vi "HW_QX_DAQ FGV.vi"(0 "DevListTree":refnum<vi>, 1 "Oper.":T3, 5 "ActiveModuTag":string, 7 "Paravalues[]":string[][](array[string]), 11 "error in":errorcluster caption="错误输入") -> (4 "ActiveCFG":T1, 6 "UsedQXcfg":T1[](array[typedef]), 8 "data":dbl[][](array[numeric]), 10 "ChanPara.CHName":string[](array[string]), 13 "SampRate":dbl, 14 "T0":timestamp, 15 "error out":errorcluster caption="错误输出")   [LabVIEW 2016]
uses:
  QX DAQ FGV Operations.ctl
  Ctrls/HardWare _ Module Configuration.ctl
panel:
  out "data":waveform(dbl)[](array[waveform])
  in  "CFGinTree":T2
  in  "QXcfg in":T1[](array[typedef])
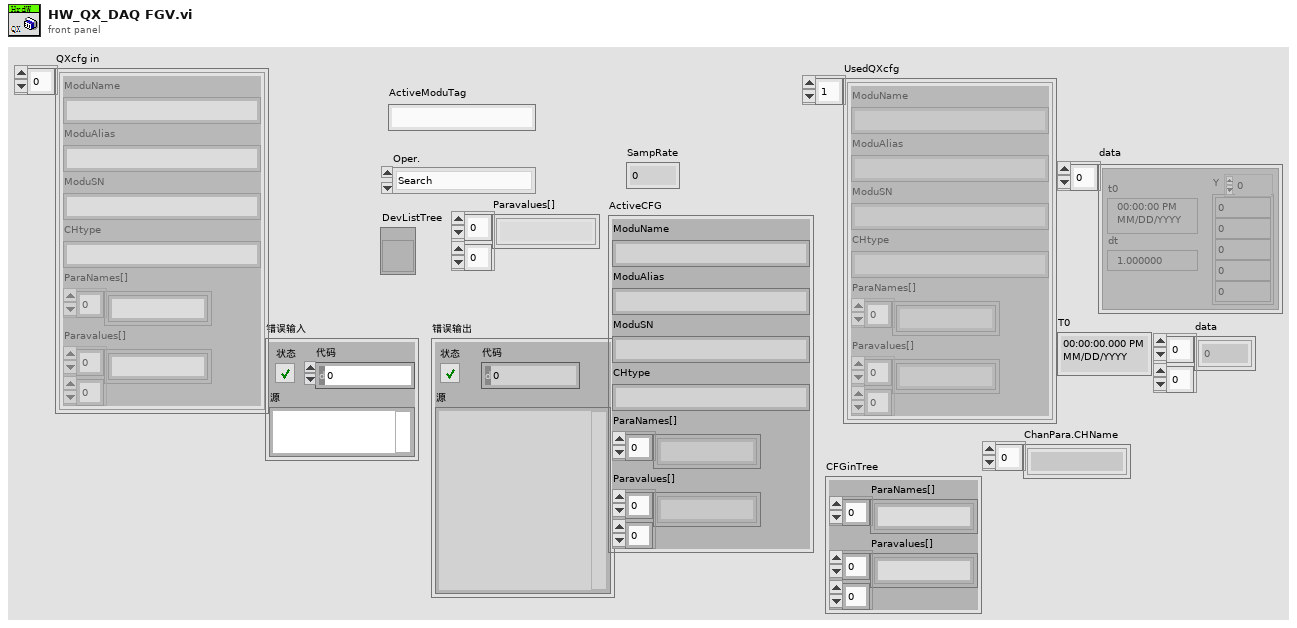
[diagram p1: front panel]
types:
  T1 = typedef "HardWare _ Module Configuration.ctl" = cluster{"ModuName":string, "ModuAlias":string, "ModuSN":string, "CHtype":string, "ParaNames[]":string[], "Paravalues[]":string[][]}
  T2 = cluster{"ParaNames[]":string[], "Paravalues[]":string[][]}
  T3 = typedef "QX DAQ FGV Operations.ctl" = enum16{"Search", "ReadCFG", "UpdateTempCFG", "DownloadCFG", "StartDAQ", "RunDAQ", "StopDAQ", "DisConnect"}
  T4 = typedef "QX Module Info.ctl" = cluster{"ModuName":string, "ModuSN":string, "ModuIP":string, "Port":i32, "ChType":string, "ChanNames[]":string[]}
  T5 = cluster{"QX DevInfo[]":T4[], "Devices":refnum<k24>[]}
  T6 = cluster{"ParaFolder":path, "SysCfg":path, "CHdef":path, "ModCfg":path, "DT Folder":path, "ErrorLog":path, "HBMDriverlicense":path}
  T7 = cluster{"ModuRef":refnum<k24>, "ChRef[]":refnum<k24>[]}[]
  T8 = typedef "HardWare _ Channel Configurations PopUp Type.ctl" = cluster{"Pop Type":T9, "PopValue":string}
  T9 = typedef "POP_Data Type.ctl" = enum16{"NO POPUP", "Unkown", "String", "Integer", "Float", "Color", "Boolean", "Ring", "Captioned String", "Captioned Integer", "Button Color", "2 Int Cluster", "4 Int Cluster", "6-Dbl Cluster", "Path", "Combox", "Time", "ShotCut String"}
  T10 = cluster{"ParaNames":string[], "DfltPara":string[], "Types":string[], "PopTypes":T8[]}
  T11 = typedef "HardWare _ Channel Parameters.ctl" = cluster{"CHType":string[], "CHName":string[], "CHAlias":string[], "Use":bool[], "Unit":string[], "SampleRate":dbl[], "FilterFreq":dbl[], "SlopeA":dbl[], "InterceptB":dbl[], "SampMax":dbl[], "SampMin":dbl[], "AlarmMax":dbl[], "AlarmMin":dbl[]}
  T12 = cluster{"AllInUsedChan[]":refnum<k24>[], "ChanPara":T11}
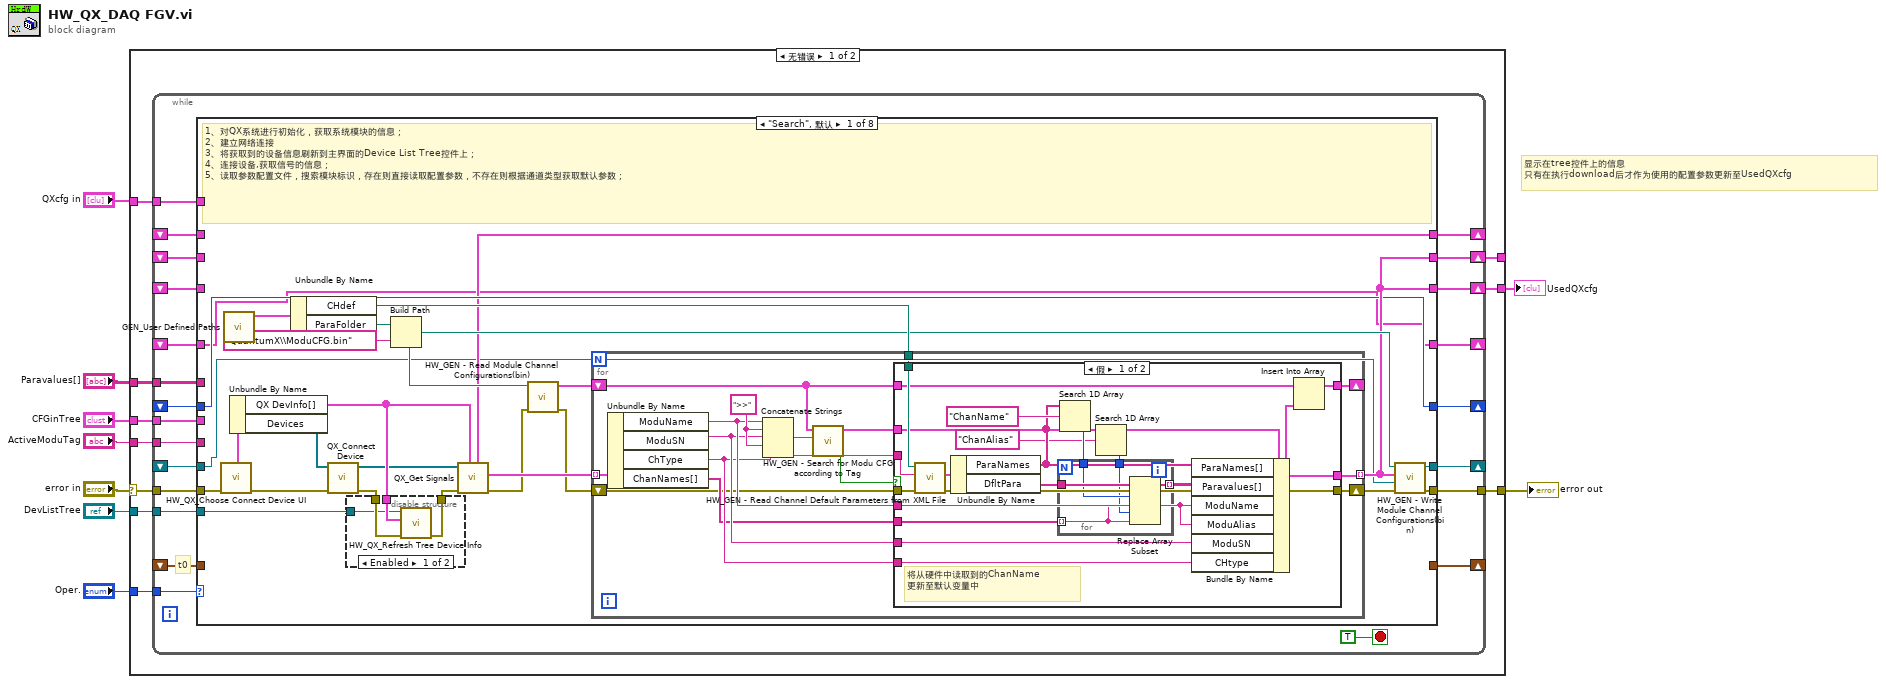
[diagram p0: block diagram]
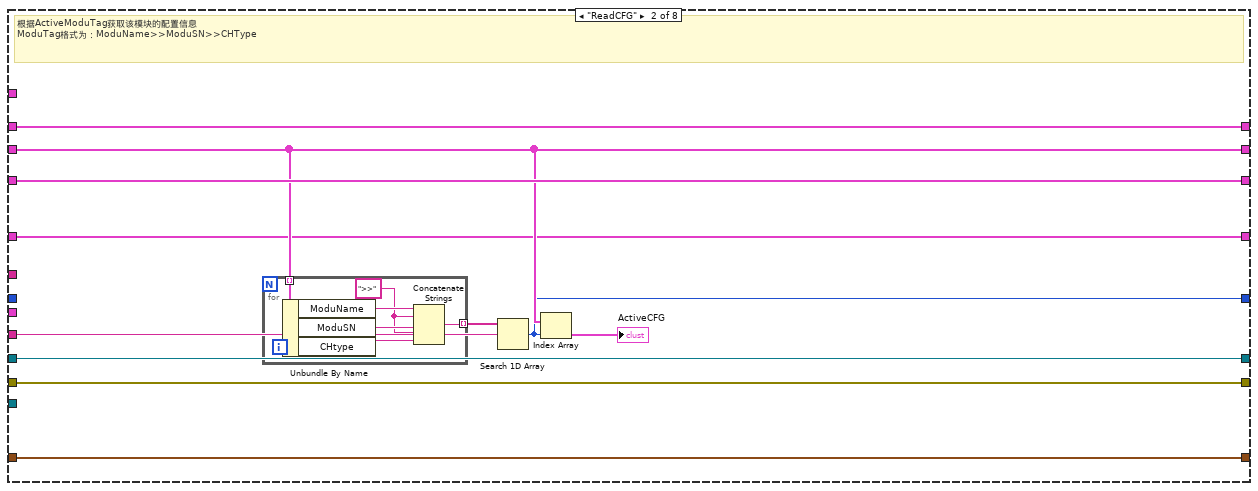
[diagram p4: hidden frame]
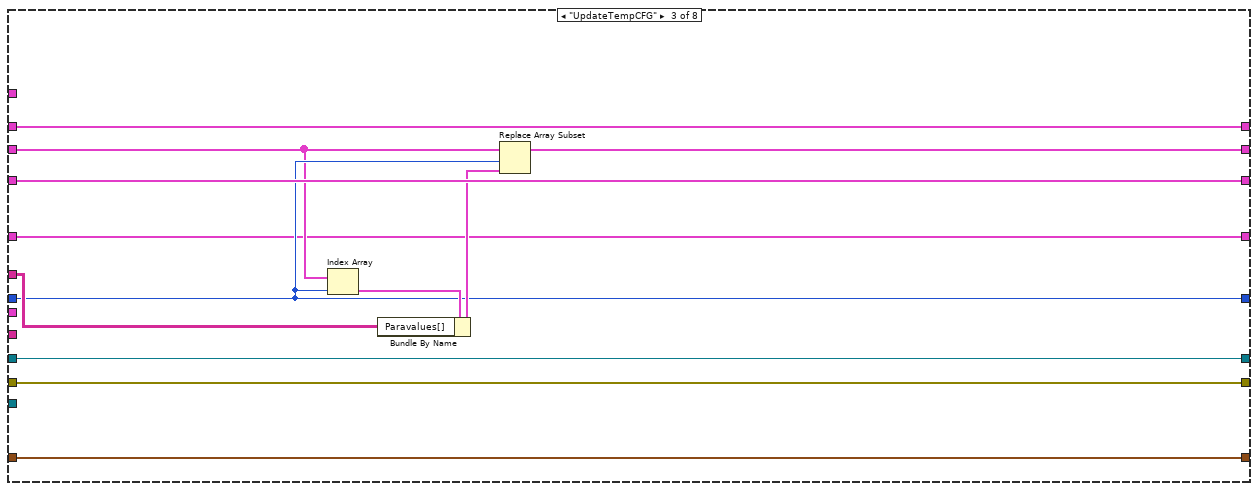
[diagram p5: hidden frame]
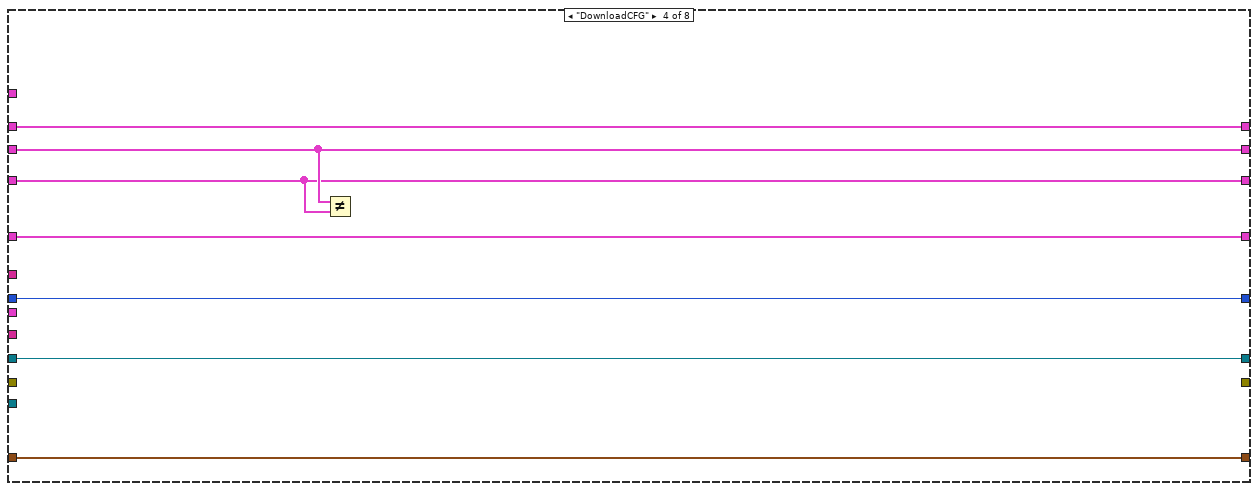
[diagram p6: hidden frame]
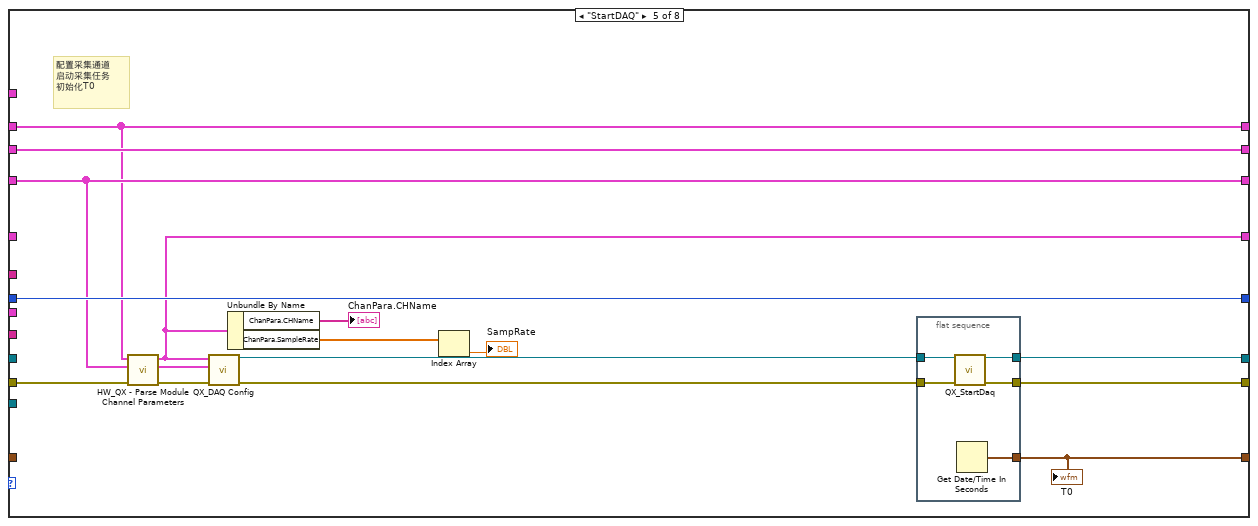
[diagram p7: hidden frame]
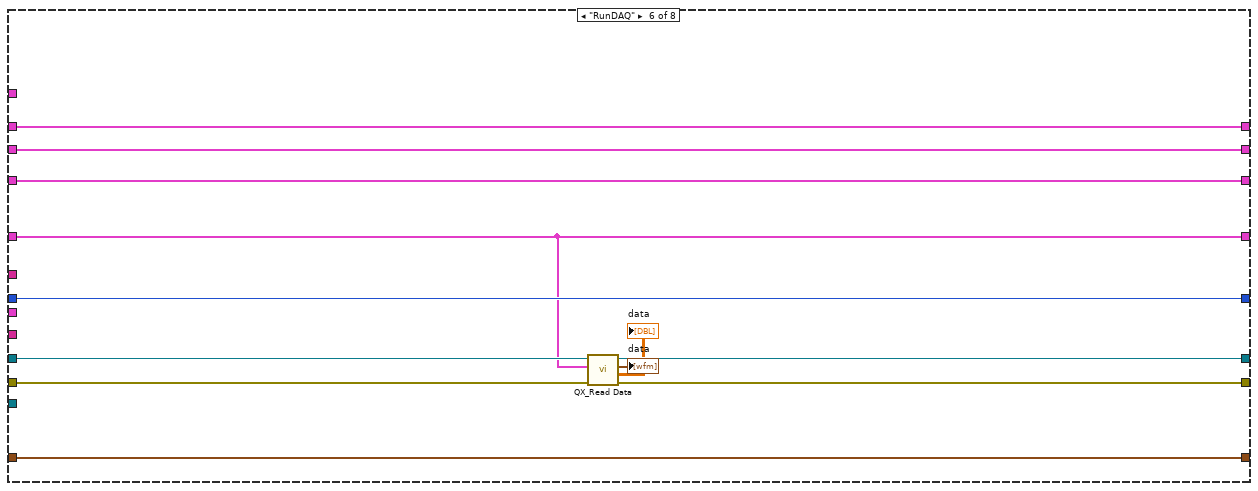
[diagram p8: hidden frame]
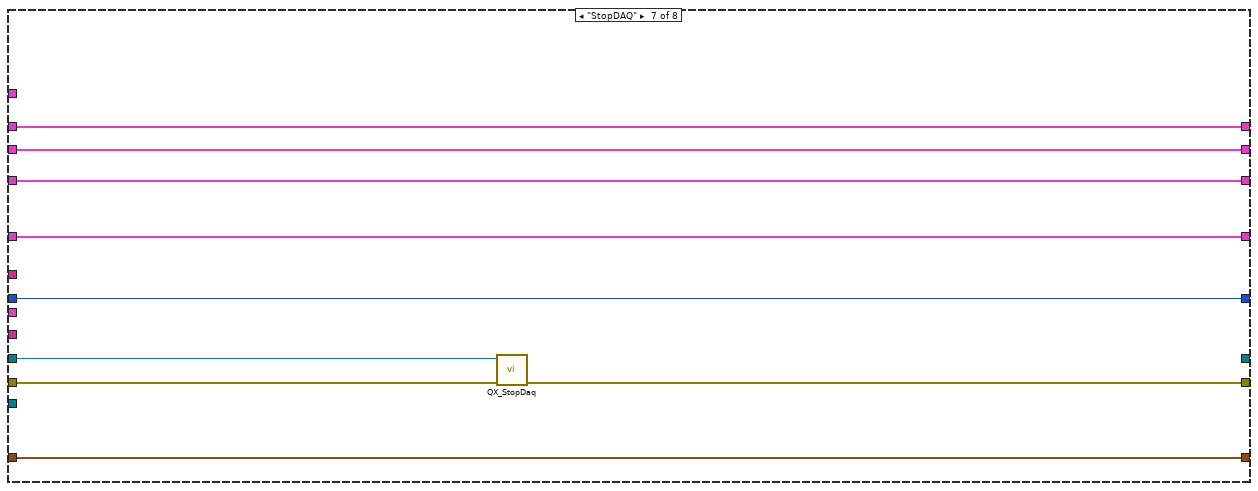
[diagram p9: hidden frame]
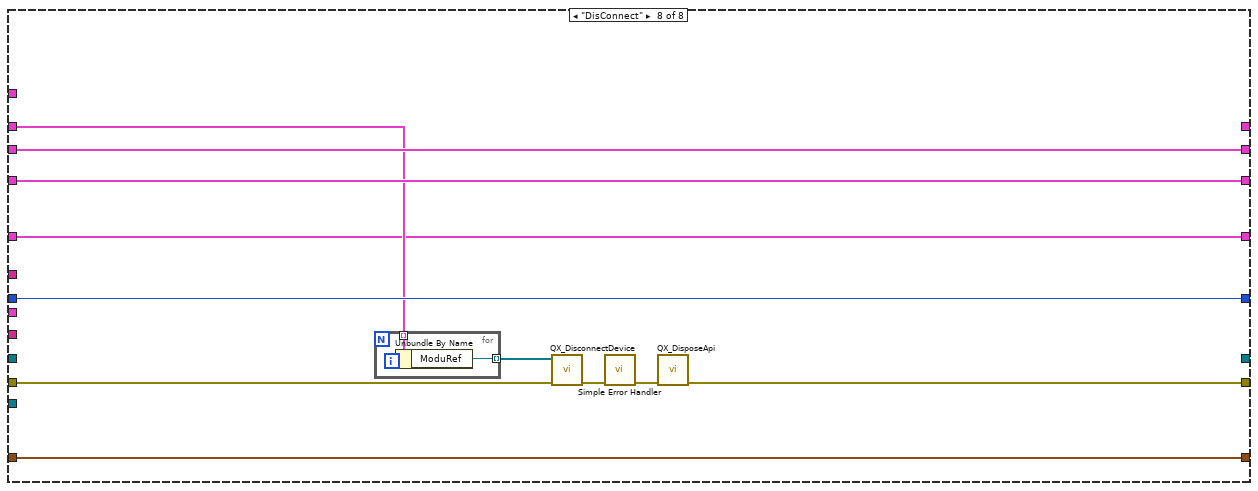
[diagram p10: hidden frame]
diagram:
  # "显示在tree控件上的信息\n只有在执行download后才作为使用的配置参数更新至UsedQXcfg"
  n1 = case shown="无错误" "error in" {
    selector: "error in" -> [w18 w207]
    tunnel: [w17 w207] -> w8
    tunnel: "Oper." -> [w19 _]
    tunnel: [w16 _] -> w6
    tunnel: "DevListTree" -> [w15 _]
    tunnel: "QXcfg in" -> [w14 _]
    tunnel: "ActiveModuTag" -> [w13 _]
    tunnel: [w12 _] -> _
    tunnel: "CFGinTree" -> [w11 _]
    tunnel: "Paravalues[]" -> [w10 _]
    frame No Error {
      n2 = while {
        tunnel: w19 -> [w41]
        tunnel: w18 -> [w40]
        tunnel: [w39] -> w17
        shift-right: [w38] -> _
        shift-left: _ -> [w37]
        shift-right: [w36] -> w16
        shift-left: _ -> [w35]
        tunnel: w15 -> [w34]
        tunnel: w14 -> [w33]
        tunnel: w13 -> [w32]
        shift-right: [w31] -> w12
        shift-left: _ -> [w30]
        tunnel: w11 -> [w29]
        shift-right: [w28] -> _
        shift-left: _ -> [w27]
        tunnel: w10 -> [w26]
        shift-right: [w25] -> _
        shift-left: _ -> [w24]
        shift-right: [w23] -> _
        shift-left: _ -> [w22]
        shift-right: [w21] -> _
        shift-left: _ -> [w20]
        stop <- TRUE stop-if-true
        # "t0"
        n3 = case shown="\"Search\", 默认" w41 {
          tunnel: w40 -> [w67 w125 w143 _ w158 w180 w187 w198]
          tunnel: [w58 w125 w143 _ w162 w177 w185 w196] -> w39
          tunnel: [_ w126 w144 w151 w167 w184 w193 w204] -> w38
          tunnel: w37 -> [_ w126 w144 w151 _ w184 w193 w204]
          tunnel: [w48 w122 w142 w145 w160 w181 w190 w203] -> w36
          tunnel: w35 -> [_ w122 w142 w145 w160 w181 w190 w203]
          tunnel: w34 -> [w53 _ _ _ _ _ _ _]
          tunnel: w33 -> [_ _ _ _ _ _ _ _]
          tunnel: w32 -> [_ w123 _ _ _ _ _ _]
          tunnel: [w48 w121 w136 w146 w165 w182 w191 w202] -> w31
          tunnel: w30 -> [_ w121 w137 w146 w165 w182 w191 w202]
          tunnel: w29 -> [_ _ _ _ _ _ _ _]
          tunnel: [w47 w120 w138 w150 w166 w183 w192 w201] -> w28
          tunnel: w27 -> [w47 _ w138 w150 w166 w183 w192 w201]
          tunnel: w26 -> [_ _ w140 _ _ _ _ _]
          tunnel: [w45 w118 w135 w149 w159 w176 w189 _] -> w25
          tunnel: w24 -> [_ w118 w135 w149 w159 w176 w189 w200]
          tunnel: [w44 w117 w134 w148 w161 w178 _ _] -> w23
          tunnel: w22 -> [w44 w117 w134 w148 _ w179 w186 _]
          tunnel: [w43 w116 w133 w147 w155 w175 w188 w194] -> w21
          tunnel: w20 -> [w43 w116 w133 w147 _ w175 w188 w194]
          frame "Search", Default {
            # "1、对QX系统进行初始化，获取系统模块的信息；\n2、建立网络连接\n3、将获取到的设备信息刷新到主界面的Device List Tree控件上；\n4、连接设备,获取信号的信息；\n5、读取参数配置文件，搜索模块标识，存在则直接读取配置参数，不存在则根据通道类型获取默认参数；"
            n4 = call "HW_QX_Choose Connect Device UI.vi"("error in"=w67) -> ("error out"=w66:errorcluster, "QX Dev"=w65:T5)  [unwired: 9 in]
            n5 = call "GEN_User Defined Paths.vi"() -> ("UserDefinedPath"=w63:T6)  [unwired: 11 in]
            n6 = Unbundle By Name(w65) -> ("QX DevInfo[]"=w54:T4[], "Devices"=w64:refnum<k24>[])
            n7 = Unbundle By Name(w63) -> ("CHdef"=w60:path, "ParaFolder"=w61:path)
            n8 = call "QX_Connect Device.vi"("error in"=w66, "Devices"=w64) -> ("error out"=w56:errorcluster, "Devices"=w46:refnum<k24>[])  [unwired: 7 in, 1 out]
            n9 = disable-structure shown="Enabled" {
              disable-tunnel: w56 -> [w71 w72]
              disable-tunnel: [w70 w72] -> w55
              disable-tunnel: w54 -> [w69 _]
              disable-tunnel: w53 -> [w68 _]
              frame Enabled {
                n10 = call "HW_QX_Refresh Tree Device Info.vi"("error in"=w71, "QXModuInfo"=w69, "Ref.Tree Ref"=w68) -> ("error out"=w70:errorcluster)  [unwired: 8 in]
              }
              frame Disabled {
              }
            }
            n11 = Build Path(base path=w61, name or relative path="QuantumX\\ModuCFG.bin") -> (appended path=w50:path)
            n12 = call "QX_Get Signals.vi"("QX Dev.QX DevInfo[]"=w54, "Error in"=w55, "ModRef[]"=w46) -> ("Error out"=w52:errorcluster, "QXModuInfo"=w57:T4[], "DevRef[]"=w45:T7)  [unwired: 6 in]
            n13 = call "HW_GEN - Read Module Channel Configurations(bin).vi"("error in"=w52, "ModuCFG path"=w50) -> ("error out"=w51:errorcluster, "ModCFG out"=w49:T1[])  [unwired: 8 in]
            n14 = for {
              tunnel: w57 -> [w84] mode=indexing
              shift-right: [w86] -> w59
              shift-left: w51 -> [w78]
              tunnel: w60 -> [w85]
              tunnel: [w79] -> w48 mode=indexing
              shift-right: [w73] -> _
              shift-left: w49 -> [w74]
              w87 = ">>" ("string")
              n15 = Unbundle By Name(w84) -> ("ModuName"=w83:string, "ModuSN"=w82:string, "ChType"=w81:string, "ChanNames[]"=w80:string[])
              n16 = Concatenate Strings(w83, w87, w82, w87, w81) -> (w77:string)
              n17 = call "HW_GEN - Search for Modu CFG according to Tag.vi"("ModuTag"=w77, "ModuCFG[]"=w74) -> ("find?"=w75:bool, "ModuCFG out"=w76:T1)  [unwired: 7 in, 1 out]
              n18 = case shown="假" w75 {
                tunnel: w78 -> [w107 w114]
                tunnel: w76 -> [w103 w115]
                tunnel: [w89 w115] -> w79
                tunnel: [w105 w114] -> w86
                tunnel: w81 -> [w106 _]
                tunnel: w85 -> [w104 _]
                tunnel: w83 -> [w102 _]
                tunnel: w82 -> [w101 _]
                tunnel: w81 -> [w100 _]
                tunnel: w80 -> [w98 _]
                tunnel: w74 -> [w90 w113]
                tunnel: [w88 w113] -> w73
                frame False {
                  # "将从硬件中读取到的ChanName\n更新至默认变量中"
                  n19 = call "HW_GEN - Read Channel Default Parameters from XML File.vi"("error in"=w107, "ChanType"=w106, "path to XML document"=w104) -> ("错误输出"=w105:errorcluster, "Chan dflt Para out"=w99:T10)  [unwired: 7 in]
                  n20 = Unbundle By Name(w99) -> ("ParaNames"=w92:string[], "DfltPara"=w97:string[])
                  n21 = Search 1D Array(1D array=w92, element="ChanName") -> (index of element=w94:i32)  [unwired: 1 in]
                  n22 = Search 1D Array(1D array=w92, element="ChanAlias") -> (index of element=w93:i32)  [unwired: 1 in]
                  n23 = for {
                    tunnel: w98 -> [w108] mode=indexing
                    tunnel: w97 -> [w112]
                    tunnel: [w111] -> w96 mode=indexing
                    tunnel: w94 -> [w110]
                    tunnel: w93 -> [w109]
                    n24 = Replace Array Subset(array=w112, new element #1=w108, index #1=w110, new element #2=w108, index #2=w109) -> (w111:string[])
                  }
                  n25 = Bundle By Name(cluster=w103, "ParaNames[]"=w92, "Paravalues[]"=w96, "ModuName"=w102, "ModuAlias"=w102, "ModuSN"=w101, "CHtype"=w100) -> (w89:T1)
                  n26 = Insert Into Array(array=w90, new element=w89) -> (w88:T1[])  [unwired: 1 in]
                }
                frame True {
                }
              }
            }
            n27 = call "HW_GEN - Write Module Channel Configurations(bin).vi"("error in"=w59, "ModuCfg"=w48, "Path"=w50) -> ("error out"=w58:errorcluster)  [unwired: 8 in]
          }
          frame "ReadCFG" {
            # "根据ActiveModuTag获取该模块的配置信息\nModuTag格式为：ModuName>>ModuSN>>CHType"
            n28 = for {
              tunnel: w121 -> [w132] mode=indexing
              tunnel: [w127] -> w124 mode=indexing
              w128 = ">>" ("string")
              n29 = Unbundle By Name(w132) -> ("ModuName"=w131:string, "ModuSN"=w130:string, "CHtype"=w129:string)
              n30 = Concatenate Strings(w131, w128, w130, w128, w129) -> (w127:string)
            }
            n31 = Search 1D Array(1D array=w124, element=w123) -> (index of element=w120:i32)  [unwired: 1 in]
            n32 = Index Array(array=w121, index=w120) -> (element=→"ActiveCFG":T1)
          }
          frame "UpdateTempCFG" {
            n33 = Index Array(array=w137, index=w138) -> (element=w141:T1)
            n34 = Bundle By Name(cluster=w141, "Paravalues[]"=w140) -> (w139:T1)
            n35 = Replace Array Subset(array=w137, new element=w139, index=w138) -> (w136:T1[])
          }
          frame "DownloadCFG" {
            n36 = Not Equal?(x=w146, y=w145) -> ()  [unwired: 1 out]
          }
          frame "StartDAQ" {
            # "配置采集通道\n启动采集任务\n初始化T0"
            n37 = call "HW_QX - Parse Module Channel Parameters.vi"("error in"=w158, "sysModCFG[]"=w160, "AllDevRef[]"=w159) -> ("error out"=w157:errorcluster, "InUsedDevRef[]"=w156:T7, "InUsedChan[]"=w155:T12)  [unwired: 6 in]
            n38 = call "QX_DAQ Config.vi"("error in"=w157, "InUsedDevRef[]"=w156, "InUsedChan[]"=w155) -> ("error out"=w164:errorcluster, "DaqMeasurement"=w163:refnum<k24>)  [unwired: 7 in]
            n39 = Unbundle By Name(w155) -> ("ChanPara.CHName"=→"ChanPara.CHName":string[], "ChanPara.SampleRate"=w153:dbl[])
            n40 = Index Array(array=w153) -> (element=→"SampRate":dbl)  [unwired: 1 in]
            n41 = flat-sequence {
              tunnel: [w172] -> w167
              tunnel: w164 -> [w171]
              tunnel: w163 -> [w170]
              tunnel: [w169] -> w162
              tunnel: [w168] -> w161
              frame #0 {
                n42 = call "QX_StartDaq.vi"("DaqMeasurement"=w170, "Error in"=w171) -> ("DaqMeasurement"=w168:refnum<k24>, "Error out"=w169:errorcluster)  [unwired: 11 in, 1 out]
                n43 = Get Date/Time In Seconds() -> (seconds since 1Jan1904=w172:timestamp)
              }
            }
            "T0" <- w167
          }
          frame "RunDAQ" {
            n44 = call "QX_Read Data.vi"("Error in"=w180, "InUsedChan[]"=w175, "DaqMeasurement"=w179) -> ("Error out"=w177:errorcluster, 1:"data"=→"data":dbl[][], 2:"data"=→"data":waveform(dbl)[], "DaqMeasurement"=w178:refnum<k24>)  [unwired: 5 in]
          }
          frame "StopDAQ" {
            n45 = call "QX_StopDaq.vi"("Error in"=w187, "DaqMeasurement"=w186) -> ("Error out"=w185:errorcluster)  [unwired: 9 in]
          }
          frame "DisConnect" {
            n46 = for {
              tunnel: w200 -> [w206] mode=indexing
              tunnel: [w205] -> w199 mode=indexing
              n47 = Unbundle By Name(w206) -> ("ModuRef"=w205:refnum<k24>)
            }
            n48 = call "QX_DisconnectDevice.vi"("Error in"=w198, "Devices"=w199) -> ("Error out"=w197:errorcluster)  [unwired: 9 in]
            n49 = call <vilib>:"Simple Error Handler.vi"("error in (no error)"=w197) -> ("error out"=w195:errorcluster)  [unwired: 4 in, 4 out]
            n50 = call "QX_DisposeApi.vi"("Error in"=w195) -> ("Error out"=w196:errorcluster)  [unwired: 10 in]
          }
        }
      }
    }
    frame Error {
    }
  }
  "error out" <- w8
  "UsedQXcfg" <- w6
